vi "Check File Permissions.vi"(8 "error in (no error)":errorcluster, 11 "path":path) -> (0 "error out":errorcluster)   [LabVIEW 2020]
doc: "Check the permission settings on the file at the specified path."
uses:
  Error Cluster From Error Code.vi
  Error Ring.xnode
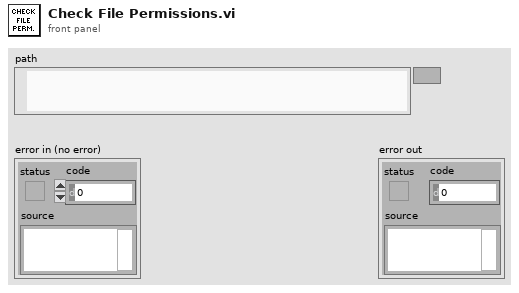
[diagram p1: front panel]
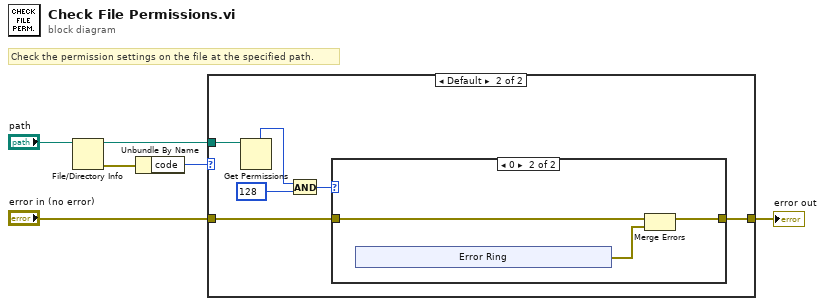
[diagram p0: block diagram]
diagram:
  # "Check the permission settings on the file at the specified path."
  n1 = File/Directory Info(path="path") -> (path out=w2:path, error out=w4:errorcluster)  [unwired: 1 in, 5 out]
  n2 = Unbundle By Name(w4) -> ("code"=w1:i32)
  n3 = case shown="Default" w1 {
    tunnel: "error in (no error)" -> [w7 w13]
    tunnel: [w7 w10] -> w3
    tunnel: w2 -> [_ w9]
    frame 7 {
    }
    frame Default {
      n4 = Get Permissions(11:w9) -> (5:w11:i16)  [unwired: 1 in, 4 out]
      n5 = And(x=w11, y=128) -> (x .and. y?=w8:i32)
      n6 = case shown="0" w8 {
        tunnel: w13 -> [w14 w17]
        tunnel: [w14 w16] -> w10
        frame Default {
        }
        frame 0 {
          n7 = xnode "Error Ring"() -> ("error out"=w15:errorcluster)
          n8 = Merge Errors(w17, w15) -> (w16:errorcluster)
        }
      }
    }
  }
  "error out" <- w3
